vi "Get Window Rectangle (hwnd).vi"(8 "error in (no error)":errorcluster, 11 "HWnd":u32) -> (0 "error out":errorcluster, 1 "Window Rect":T1, 3 "HWnd Out":u32)   [LabVIEW 2011]
doc: "This VI will find the coordinates of the upper left and lower right corners of the window identified by the 'window refnum' parameter. Coordinate values are in pixels, relative to the upper left corner of the screen. The 'window refnum' can be obtained by using 'Get Window RefNum.vi'."
uses:
  Controls/Window Rectangle (hwnd).ctl
  user32.dll
  kernel32.dll
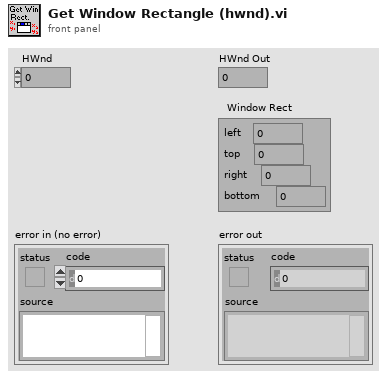
[diagram p1: front panel]
types:
  T1 = typedef "Window Rectangle (hwnd).ctl" = cluster{"left":i16, "top":i16, "right":i16, "bottom":i16}
  T2 = cluster{"RECT[0]":i32, "RECT[1]":i32, "RECT[2]":i32, "RECT[3]":i32}
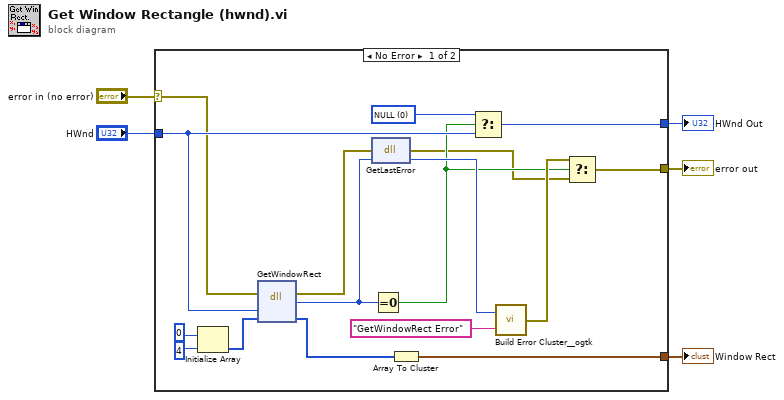
[diagram p0: block diagram]
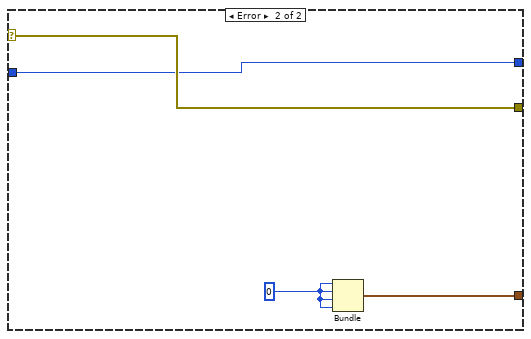
[diagram p2: hidden frame]
diagram:
  n1 = case shown="No Error" "error in (no error)" {
    selector: "error in (no error)" -> [w13 w24]
    tunnel: [w22 w23] -> w3
    tunnel: [w6 w24] -> w1
    tunnel: "HWnd" -> [w14 w23]
    tunnel: [w17 w26] -> w5
    frame No Error {
      w15 = u32 0 items=["NULL"]
      n2 = Initialize Array(0, 4) -> (w19:i32[])
      n3 = dll-call lib="USER32.DLL" fn="GetWindowRect"(error in=w13, "hWnd"=w14, "RECT"=w19) -> (error out=w12:errorcluster, "Return Value"=w16:i32, "RECT"=w18:i32[])  [unwired: 3 in, 1 out]
      n4 = dll-call lib="kernel32.dll" fn="GetLastError"(error in=w12, w16) -> (error out=w7:errorcluster, w9:i32)  [unwired: 1 in, 1 out]
      n5 = Equal To 0?(x=w16) -> (x = 0?=w8:bool)
      n6 = Array To Cluster(array=w18) -> (cluster=w17:T2)
      n7 = Select(t=w15, s=w8, f=w14) -> (s? t:f=w22:u32)
      n8 = call <userlib>:"Build Error Cluster__ogtk.vi"("String to Prepend to source (\"\")"="GetWindowRect Error" ("String to Prepend to source (\"\")"), "code"=w9) -> ("error out"=w10:errorcluster)
      n9 = Select(t=w10, s=w8, f=w7) -> (s? t:f=w6:errorcluster)
    }
    frame Error {
      w25 = i16 0
      n10 = Bundle(w25, w25, w25, w25) -> (w26:cluster{i16, i16, i16, i16})  [unwired: 1 out]
    }
  }
  "Window Rect" <- w5
  "error out" <- w1
  "HWnd Out" <- w3
